vi "Error Process.vi"(8 "error in (no error)":errorcluster, 10 "Queues":T1, 11 "UE Data Container":T2) -> (0 "error out":errorcluster)   [LabVIEW 2017]
doc: "Centrilized Error Handler of ATM controller"
uses:
  Shared Data/User Events/UE Data Container.ctl
  Controls/Error Data.ctl
  UIs/User Console/Controls/User Console - Transaction Enum.ctl
  Shared Data/Queues/Controls/Queues.ctl
  Controller/Controls/Controller CMD.ctl
  Configuration/Controls/Config CMD.ctl
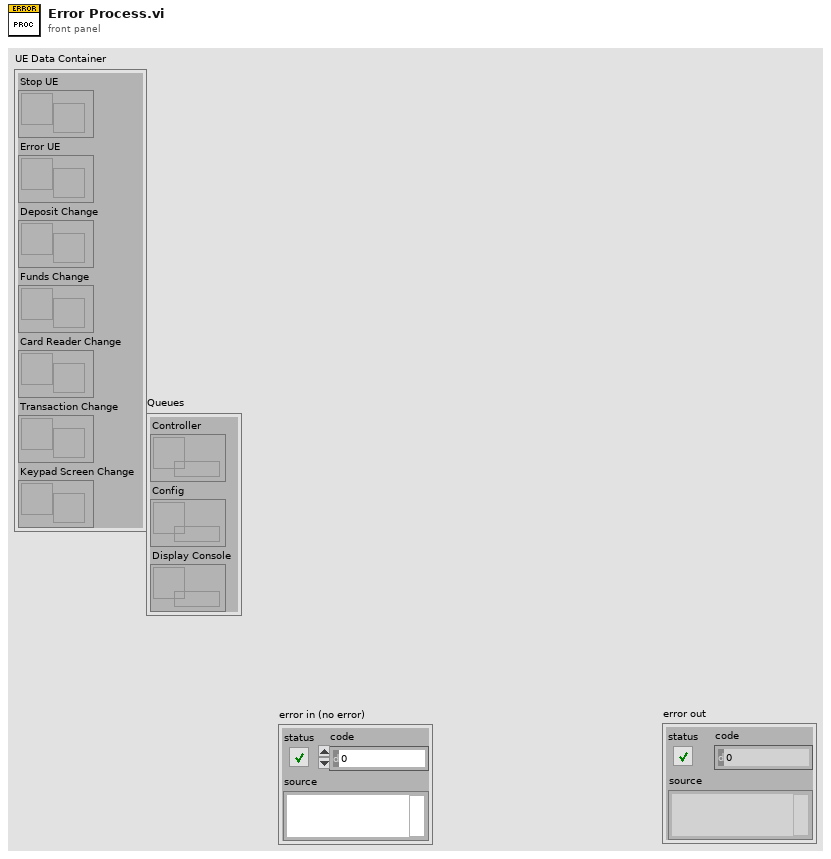
[diagram p1: front panel]
types:
  T1 = typedef "Queues.ctl" = cluster{"Controller":refnum<queue>, "Config":refnum<queue>, "Display Console":refnum<queue>}
  T2 = typedef "UE Data Container.ctl" = cluster{"Stop UE":refnum<user-event>, "Error UE":refnum<user-event>, "Deposit Change":refnum<user-event>, "Funds Change":refnum<user-event>, "Card Reader Change":refnum<user-event>, "Transaction Change":refnum<user-event>, "Keypad Screen Change":refnum<user-event>}
  T3 = typedef "Controller CMD.ctl" = cluster{"Command":enum16{"Idle", "Init", "Config Update", "Terminate", "Send Message", "Login Start", "Login Finish", "Balance", "Deposit", "Withdrawal", "Fast Cash Start", "Fast Cash Stop", "Keypad Proc", "Search Account"}, "Data":variant}
  T4 = typedef "Error Data.ctl" = cluster{"Type":enum16{"Console Error", "Sensor Interface IO Error", "Process Step Error"}, "Data":variant}
  T5 = enum16{"Console Error", "Sensor Interface IO Error", "Process Step Error"}
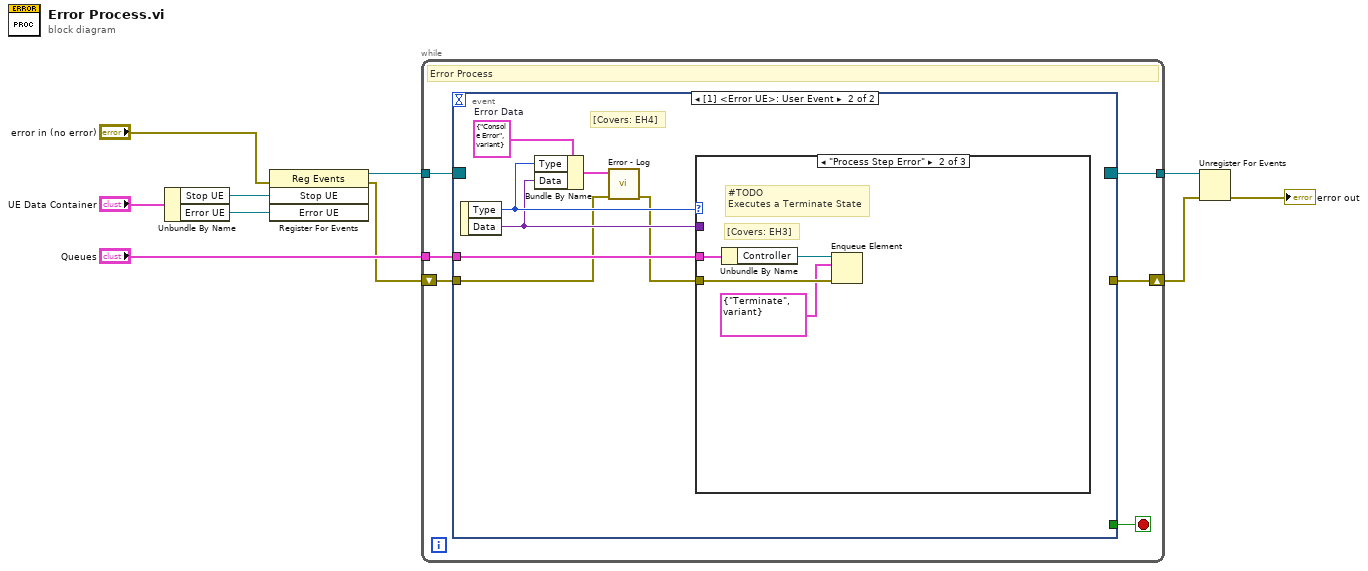
[diagram p0: block diagram]
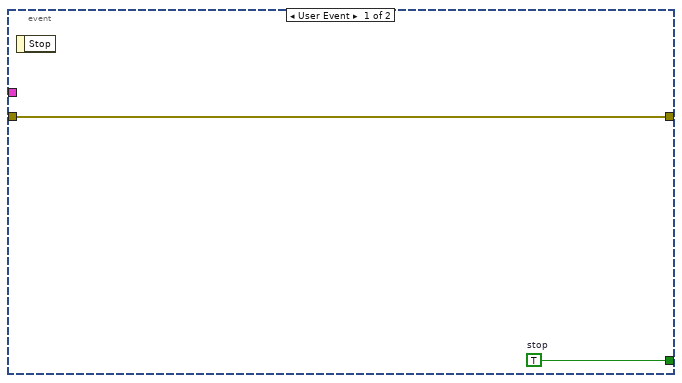
[diagram p2: hidden frame]
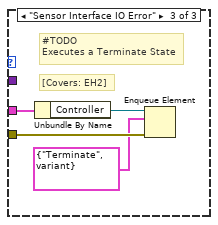
[diagram p4: hidden frame]
diagram:
  n1 = Unbundle By Name("UE Data Container") -> ("Stop UE"=w9:refnum<user-event>, "Error UE"=w1:refnum<user-event>)
  n2 = register-events(error in="error in (no error)", w9, w1) -> (reference out=w7:refnum<event-registration>, error out=w3:errorcluster)  [unwired: 1 in]
  n3 = while {
    tunnel: w7 -> [w16]
    tunnel: [w15] -> w6
    tunnel: "Queues" -> [w13]
    shift-right: [w11] -> w5
    shift-left: w3 -> [w12]
    stop <- w14 stop-if-true
    # "Error Process"
    n4 = event shown="[1] <Error UE>: User Event" {
      selector: w16 -> [_ _]
      dyn-events: [_ _] -> w15
      timeout: _ -> [_ _]
      tunnel: [w18 _] -> w14
      tunnel: w13 -> [_ w25]
      tunnel: w12 -> [w17 w20]
      tunnel: [w17 _] -> w11
      event User Event {
        w18 = TRUE  # stop
        n5 = event-data() -> ()  [unwired: 1 in, 1 out]
      }
      event User Event {
        w24 = T4 {"Type"=enum."Console Error", "Data"=variant}  # Error Data
        # "[Covers: EH4]"
        n6 = event-data() -> ("Type"=w23:T5, "Data"=w22:variant)  [unwired: 1 in]
        n7 = Bundle By Name(cluster=w24, "Type"=w23, "Data"=w22) -> (w21:T4)
        n8 = call "Error - Log.vi"("error in (no error)"=w20, "Error Data"=w21) -> ("error out"=w19:errorcluster)  [unwired: 9 in]
        n9 = case shown="\"Process Step Error\"" w23 {
          tunnel: w22 -> [_ _ _]
          tunnel: w25 -> [_ w29 w33]
          tunnel: w19 -> [_ w27 w31]
          frame "Console Error", Default {
            # "[Covers: EH1B2]"
            # "[Covers: EH1B1]"
            # "[Covers: EH1B]"
            # "[Covers: EH1A]"
            # "#TODO\nCheck a source of Error\nIF Error source = Display Console \nTHEN displays notification dialog to user AND after OK continue \nlast operation.\nIF Error source = User Console\nTHEN displays dialog to user with Clear and Continue buttons\n  IF user press Clear THEN continue last operation\n  ELSE handle Error as Process Step Error\n\nError source get from variant Data"
            # "[Covers: EH1]"
            # "#TODO\nNotify user about the error and continue ATM operations\nwithout interruption"
          }
          frame "Process Step Error" {
            # "[Covers: EH3]"
            # "#TODO\nExecutes a Terminate State"
            n10 = Unbundle By Name(w29) -> ("Controller"=w28:refnum<queue>)
            n11 = Enqueue Element(queue=w28, element=T3 {"Command"=enum."Terminate", "Data"=variant} ("Controller CMD"), error in (no error)=w27) -> ()  [unwired: 1 in, 3 out]
          }
          frame "Sensor Interface IO Error" {
            # "[Covers: EH2]"
            # "#TODO\nExecutes a Terminate State"
            n12 = Unbundle By Name(w33) -> ("Controller"=w32:refnum<queue>)
            n13 = Enqueue Element(queue=w32, element=T3 {"Command"=enum."Terminate", "Data"=variant} ("Controller CMD"), error in (no error)=w31) -> ()  [unwired: 1 in, 3 out]
          }
        }
      }
    }
  }
  n14 = Unregister For Events(event registration refnum=w6, error in=w5) -> (error out=→"error out":errorcluster)
